vi "Move Axis.vi"(3 "Make Vertical":bool, 4 "Side":T1=enum."right", 5 "Label":string, 6 "Wait Time":dbl, 8 "error in":errorcluster, 9 "Speed":dbl=25.0, 10 "Value":dbl, 11 "Location":string="Z") -> (0 "error out":errorcluster)   [LabVIEW 2013]
uses:
  ROS/Code/SubVIs/BaxterSide.ctl
  ROS/Code/Console/Servers/ServerSubs/(nist) Arm Globals.vi
  Prim/Fwd Kenimatics - array.vi
  Move Matrix.vi
  <vilib>/Analysis/Matrix/Numeric/Multiply/Multiply - RM,RM.vi
  <vilib>/Analysis/Matrix/NI_Matrix.lvlib
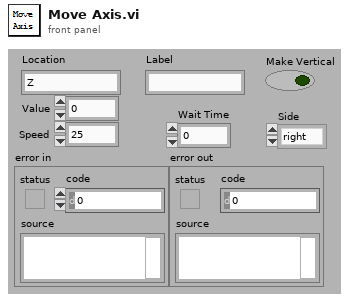
[diagram p1: front panel]
types:
  T1 = typedef "BaxterSide.ctl" = enum16{"left", "right"}
  T2 = typedef "NI_Matrix.lvlib/RealMatrix.ctl" = dbl[][]
  T3 = cluster{"X":dbl, "Y":dbl, "Z":dbl, "Roll":dbl, "Pitch":dbl, "Yaw":dbl}
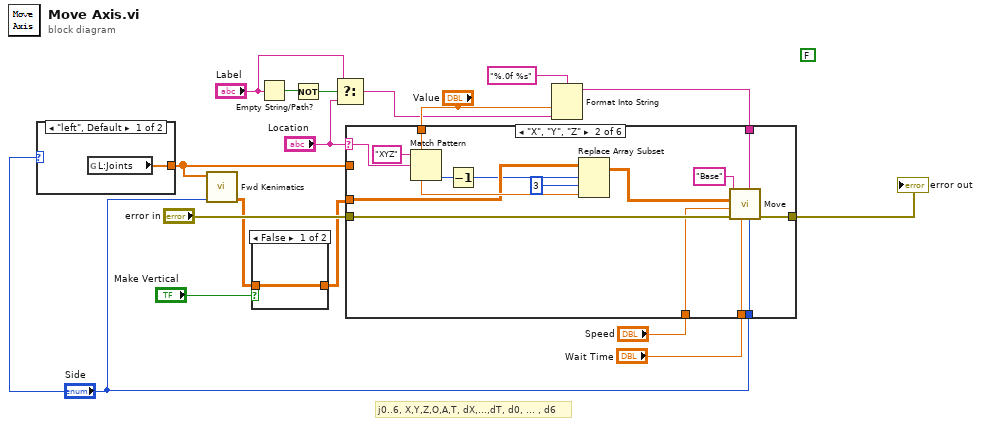
[diagram p0: block diagram]
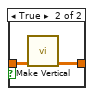
[diagram p2: hidden frame]
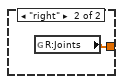
[diagram p3: hidden frame]
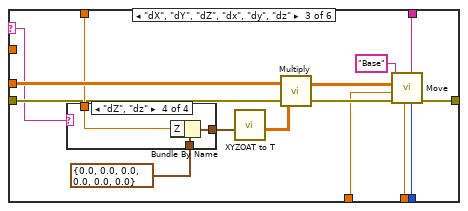
[diagram p5: hidden frame]
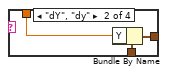
[diagram p7: hidden frame]
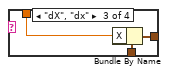
[diagram p8: hidden frame]
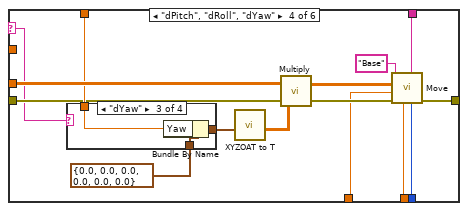
[diagram p9: hidden frame]
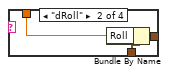
[diagram p11: hidden frame]
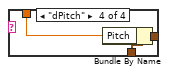
[diagram p12: hidden frame]
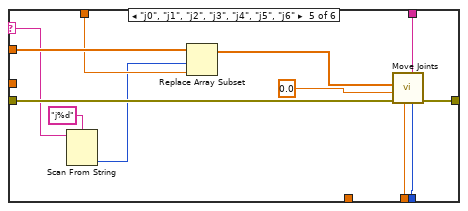
[diagram p13: hidden frame]
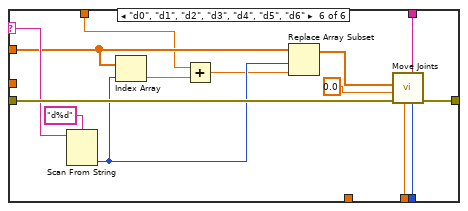
[diagram p14: hidden frame]
diagram:
  (unwired) FALSE ("Relative")
  # "j0..6, X,Y,Z,O,A,T, dX,...,dT, d0, ... , d6"
  n1 = case shown="\"left\", Default" "Side" {
    tunnel: [w18 w19] -> w9
    frame "left", Default {
      n2 = global read "(nist) Arm Globals.vi" "L:Joints"() -> (w18:dbl[])
    }
    frame "right" {
      n3 = global read "(nist) Arm Globals.vi" "R:Joints"() -> (w19:dbl[])
    }
  }
  n4 = call-poly "Fwd Kenimatics.vi"("Side"="Side", "Joints"=w9) -> ("Matrix"=w3:T2)  [unwired: 8 in, 1 out]
  n5 = case shown="False" "Make Vertical" {
    tunnel: w3 -> [w20 w22]
    tunnel: [w20 w21] -> w2
    frame False {
    }
    frame True {
      n6 = call "Make Vertical.vi"("Matrix"=w22) -> ("Vertical Matrix"=w21:T2)  [unwired: 10 in]
    }
  }
  n7 = Empty String/Path?(string/path="Label") -> (empty?=w8:bool)
  n8 = Not(x=w8) -> (.not. x?=w7:bool)
  n9 = Select(t="Label", s=w7, f="Location") -> (s? t:f=w5:string)
  n10 = Format Into String(format string="%.0f %s" ("Label"), "Value", w5) -> (resulting string=w15:string)  [unwired: 2 in, 1 out]
  n11 = case shown="\"X\", \"Y\", \"Z\"" "Location" {
    selector: "Location" -> [_ w29 w41 w65 w92 w108]
    tunnel: "Value" -> [_ w37 w48 w72 w97 w103]
    tunnel: w2 -> [_ w36 w49 w73 _ _]
    tunnel: w9 -> [_ _ _ _ w98 w106]
    tunnel: "Side" -> [_ w25 w40 w63 w88 w100]
    tunnel: w15 -> [_ w33 w43 w67 w89 w101]
    tunnel: "error in" -> [w23 w32 w46 w70 w93 w109]
    tunnel: [w23 w31 w42 w66 w94 w110] -> w14
    tunnel: "Speed" -> [_ w30 w44 w68 _ _]
    tunnel: "Wait Time" -> [_ w24 w39 w64 w87 w99]
    frame Default {
    }
    frame "X", "Y", "Z" {
      n12 = Match Pattern(string="XYZ", regular expression=w29) -> (offset past match=w27:i32)  [unwired: 1 in, 3 out]
      n13 = Decrement(x=w27) -> (x-1=w26:i32)
      n14 = Replace Array Subset(array=w36, new element=w37, index (row)=w26, index (col)=3 ("disabled index (row)")) -> (w35:T2)
      n15 = call-poly "Move.vi"("Side"=w25, "Label"=w33, "Wait Time"=w24, "error in"=w32, "Speed (mm/s)"=w30, "Offset"=w35, "Location"="Base") -> ("error out"=w31:errorcluster)  [unwired: 4 in]
    }
    frame "dX", "dY", "dZ", "dx", "dy", "dz" {
      n16 = case shown="\"dZ\", \"dz\"" w41 {
        tunnel: [w53 w56 w59 w62] -> w52
        tunnel: T3 {"X"=0.0, "Y"=0.0, "Z"=0.0, "Roll"=0.0, "Pitch"=0.0, "Yaw"=0.0} ("XYZOAT") -> [w53 w55 w58 w61]
        tunnel: w48 -> [_ w54 w57 w60]
        frame Default {
        }
        frame "dY", "dy" {
          n17 = Bundle By Name(cluster=w55, "Y"=w54) -> (w56:T3)
        }
        frame "dX", "dx" {
          n18 = Bundle By Name(cluster=w58, "X"=w57) -> (w59:T3)
        }
        frame "dZ", "dz" {
          n19 = Bundle By Name(cluster=w61, "Z"=w60) -> (w62:T3)
        }
      }
      n20 = call "XYZOAT to T.vi"("XYZOAT"=w52) -> ("T"=w50:T2)  [unwired: 10 in]
      n21 = call-poly <vilib>:"Multiply.vi"("Real Matrix B"=w50, "Real Matrix A"=w49) -> ("A * B"=w45:T2)
      n22 = call-poly "Move.vi"("Side"=w40, "Label"=w43, "Wait Time"=w39, "error in"=w46, "Speed (mm/s)"=w44, "Offset"=w45, "Location"="Base") -> ("error out"=w42:errorcluster)  [unwired: 4 in]
    }
    frame "dPitch", "dRoll", "dYaw" {
      n23 = case shown="\"dYaw\"" w65 {
        tunnel: [w77 w80 w83 w86] -> w76
        tunnel: T3 {"X"=0.0, "Y"=0.0, "Z"=0.0, "Roll"=0.0, "Pitch"=0.0, "Yaw"=0.0} ("XYZOAT") -> [w77 w79 w82 w85]
        tunnel: w72 -> [_ w78 w81 w84]
        frame Default {
        }
        frame "dRoll" {
          n24 = Bundle By Name(cluster=w79, "Roll"=w78) -> (w80:T3)
        }
        frame "dYaw" {
          n25 = Bundle By Name(cluster=w82, "Yaw"=w81) -> (w83:T3)
        }
        frame "dPitch" {
          n26 = Bundle By Name(cluster=w85, "Pitch"=w84) -> (w86:T3)
        }
      }
      n27 = call "XYZOAT to T.vi"("XYZOAT"=w76) -> ("T"=w74:T2)  [unwired: 10 in]
      n28 = call-poly <vilib>:"Multiply.vi"("Real Matrix B"=w74, "Real Matrix A"=w73) -> ("A * B"=w69:T2)
      n29 = call-poly "Move.vi"("Side"=w63, "Label"=w67, "Wait Time"=w64, "error in"=w70, "Speed (mm/s)"=w68, "Offset"=w69, "Location"="Base") -> ("error out"=w66:errorcluster)  [unwired: 4 in]
    }
    frame "j0", "j1", "j2", "j3", "j4", "j5", "j6" {
      n30 = Scan From String(format string="j%d", input string=w92) -> (output 1=w90:i32)  [unwired: 3 in, 3 out]
      n31 = Replace Array Subset(array=w98, new element=w97, index=w90) -> (w96:dbl[])
      n32 = call "Move Joints.vi"("Side"=w88, "Label"=w89, "Wait (s)"=w87, "error in"=w93, "time"=0.0, "Goal"=w96) -> ("error out"=w94:errorcluster)  [unwired: 4 in, 1 out]
    }
    frame "d0", "d1", "d2", "d3", "d4", "d5", "d6" {
      n33 = Scan From String(format string="d%d", input string=w108) -> (output 1=w105:i32)  [unwired: 3 in, 3 out]
      n34 = Index Array(array=w106, index=w105) -> (element=w104:dbl)
      n35 = Add(x=w103, y=w104) -> (x+y=w102:dbl)
      n36 = Replace Array Subset(array=w106, new element=w102, index=w105) -> (w112:dbl[])
      n37 = call "Move Joints.vi"("Side"=w100, "Label"=w101, "Wait (s)"=w99, "error in"=w109, "time"=0.0, "Goal"=w112) -> ("error out"=w110:errorcluster)  [unwired: 4 in, 1 out]
    }
  }
  "error out" <- w14
